vi "Test Launch For Nested Actor Without Caller.vi"(4 "Debug Alias (\"\")":string, 6 "Open Actor Core front panel? (F)":bool, 8 "error in (no error)":errorcluster, 9 "timeout in ms (-1)":i32=-1, 11 "Actor Before Launch":refnum<class "Actor.lvclass">) -> (0 "error out":errorcluster, 3 "Actor After Stop":refnum<class "Actor.lvclass">)   [LabVIEW 2020]
doc: "Often you want to test a nested actor's behaviors without spinning up your full actor tree. You can write a test harness actor to use as a caller that will launch your nested actor, send it various test messages and monitor it for responses. Then you have to launch that test harness actor and somehow get the test results out of it. This VI allows you to easily get those test results. You pass an unlaunched test harness actor in and this VI sychronously launches and waits for the stop of that actor and returns to you the actor in its final state.\n\nYou can supply a <b>timeout in ms</b>. If the actor takes too long to run, it will be stopped with an Emergency Stop message; this VI will return error code 1639 indicating that a timeout occurred."
uses:
  Actor/Actor.lvclass
  Message Queue/Message Queue.lvclass/Message Queue.ctl
  Message Dequeuer/Message Dequeuer.lvclass/Message Dequeuer.ctl
  LastAck/Last Ack.lvclass
  LastAck/Last Ack.lvclass/Last Ack.ctl
  Stop Msg/Stop Msg.lvclass/Stop Msg.ctl
  Message Enqueuer/Message Enqueuer.lvclass/Message Enqueuer.ctl
  Message Enqueuer/Enqueue Critical.vi
  Stop Msg/Stop Msg.lvclass
  C:/justACS/Actor Framework/Core/ActorFramework/Message/Message.lvclass
  Message Priority Queue/Priority Dequeue.vi
  Message Priority Queue/Priority Enqueue.vi
  <vilib>/Utility/error.llb/Error Cluster From Error Code.vi
  <vilib>/ErrorRing/Error Ring.xnode
  Message Queue/Message Queue.lvclass
  Message Dequeuer/Message Dequeuer.lvclass
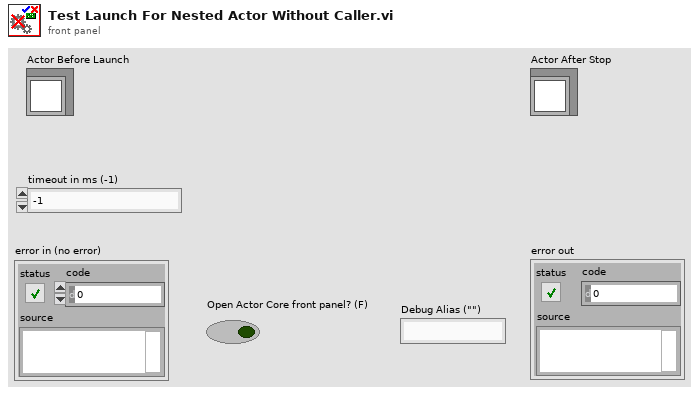
[diagram p1: front panel]
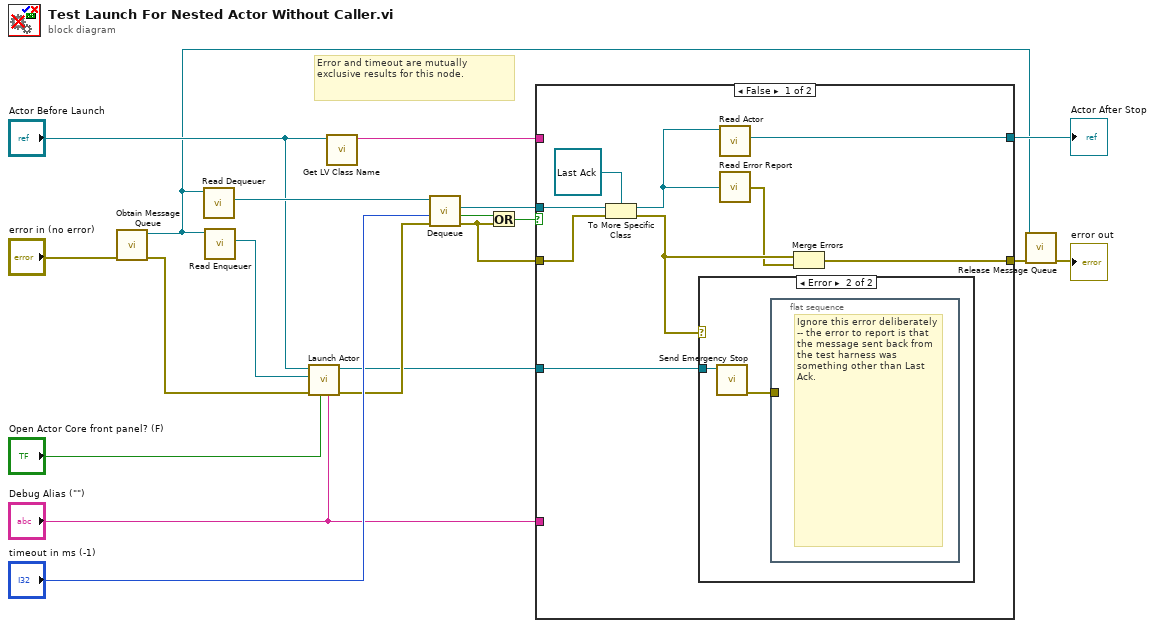
[diagram p0: block diagram]
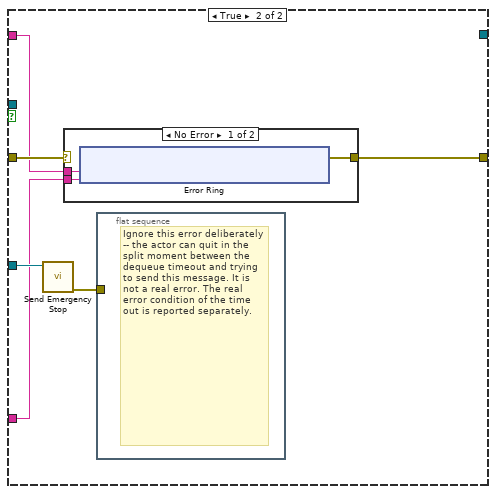
[diagram p3: hidden frame]
diagram:
  # "Error and timeout are mutually exclusive results for this node."
  n1 = call "Obtain Message Queue.vi"("error in (no error)"="error in (no error)") -> ("error out"=w18:errorcluster, "Message Queue"=w1:refnum<class "Message Queue.lvclass">)  [unwired: 9 in]
  n2 = call "Read Dequeuer.vi"("Message Queue"=w1) -> ("Message Dequeuer"=w16:refnum<class "Message Dequeuer.lvclass">)  [unwired: 10 in]
  n3 = call "Read Enqueuer.vi"("Message Queue"=w1) -> ("Message Enqueuer"=w19:refnum<class "Message Enqueuer.lvclass">)  [unwired: 10 in]
  n4 = call "Launch Actor.vi"("Debug Alias"="Debug Alias (\"\")", "Open Actor Core front panel? (F)"="Open Actor Core front panel? (F)", "error in (no error)"=w18, "Actor-to-Caller Enqueuer"=w19, "Actor"="Actor Before Launch") -> ("error out"=w14:errorcluster, "Caller-To-Actor Enqueuer"=w12:refnum<class "Message Enqueuer.lvclass">)  [unwired: 5 in]
  n5 = call <vilib>:"Get LV Class Name.vi"("object"="Actor Before Launch") -> ("class name"=w7:string)  [unwired: 9 in, 1 out]
  n6 = call "Dequeue.vi"("error in (no error)"=w14, "timeout in ms (-1)"="timeout in ms (-1)", "Message Dequeuer in"=w16) -> ("error out"=w9:errorcluster, "timed out?"=w11:bool, "Message"=w13:refnum<class "Message.lvclass">)  [unwired: 4 in, 2 out]
  n7 = Or(x=w11, y=w9) -> (x .or. y?=w10:bool)
  n8 = case shown="False" w10 {
    tunnel: w13 -> [w28 _]
    tunnel: w12 -> [w25 w36]
    tunnel: w9 -> [w26 w34]
    tunnel: [w21 w33] -> w6
    tunnel: w7 -> [_ w32]
    tunnel: [w20 _] -> w4
    tunnel: "Debug Alias (\"\")" -> [_ w31]
    frame False {
      n9 = To More Specific Class(target class=refnum<class "Last Ack.lvclass"> refnum ("Last Ack"), reference=w28, error in=w26) -> (specific class reference=w24:refnum<class "Last Ack.lvclass">, error out=w23:errorcluster)
      n10 = case shown="Error" w23 {
        tunnel: w25 -> [_ w29]
        frame No Error {
        }
        frame Error {
          n11 = call "Send Emergency Stop.vi"("Message Enqueuer"=w29) -> ("error out"=w30:errorcluster)  [unwired: 10 in]
          n12 = flat-sequence {
            tunnel: w30 -> [_]
            frame #0 {
              # "Ignore this error deliberately -- the error to report is that the message sent back from the test harness was something other than Last Ack."
            }
          }
        }
      }
      n13 = call "Read Actor.vi"("Last Ack"=w24) -> ("Actor"=w20:refnum<class "Actor.lvclass">)  [unwired: 10 in]
      n14 = call "Read Error Report.vi"("Last Ack"=w24) -> ("error report"=w22:errorcluster)
      n15 = Merge Errors(w23, w22) -> (w21:errorcluster)
    }
    frame True {
      n16 = call "Send Emergency Stop.vi"("Message Enqueuer"=w36) -> ("error out"=w35:errorcluster)  [unwired: 10 in]
      n17 = case shown="No Error" w34 {
        selector: w34 -> [_ w48]
        tunnel: [w38 w48] -> w33
        tunnel: w32 -> [w39 _]
        tunnel: w31 -> [w37 _]
        frame No Error {
          n18 = xnode "Error Ring"("parameter 0"=w39, "parameter 1"=w37) -> ("error out"=w38:errorcluster)
        }
        frame Error {
        }
      }
      n19 = flat-sequence {
        tunnel: w35 -> [_]
        frame #0 {
          # "Ignore this error deliberately -- the actor can quit in the split moment between the dequeue timeout and trying to send this message. It is not a real error. The real error condition of the time out is reported separately."
        }
      }
    }
  }
  "Actor After Stop" <- w4
  n20 = call "Release Message Queue.vi"("error in (no error)"=w6, "Message Queue"=w1) -> ("error out"=→"error out":errorcluster)  [unwired: 8 in, 1 out]
